vi "PublicAlarms.vi"(0 "reference in":refnum<class "Logger.lvclass">, 11 "error in (no error)":errorcluster, 13 "SV_Publisher in":refnum<class "SV_Publisher.lvclass">) -> (4 "reference out":refnum<class "Logger.lvclass">, 15 "error out":errorcluster)   [LabVIEW 2019, in "Logger.lvclass"]
uses:
  Logger.lvclass
  SV_Puplisher_class/SV_Publisher.lvclass
  Current Alarms.ctl
  EventData.ctl
  TypeDef/AlarmType.ctl
  Logger.lvclass/Logger.ctl
  SV_Puplisher_class/SV_Publisher.lvclass/SV_Publisher.ctl
  SV_Puplisher_class/Set SV.vi/1ae5d02c-efd0-450a-8aa4-8388e25d05bc.vi
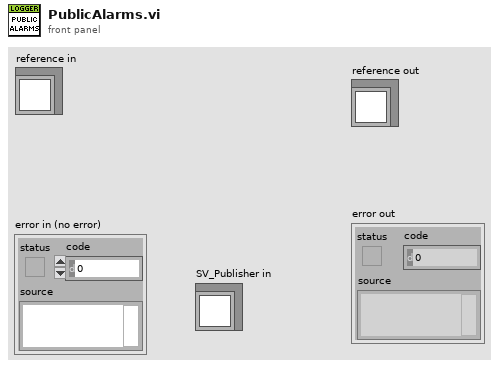
[diagram p1: front panel]
types:
  T1 = typedef "Logger.lvclass/Current Alarms.ctl" = cluster{"alarms":T2[]}
  T2 = typedef "Logger.lvclass/EventData.ctl" = cluster{"obj_tag":string, "event_tag":string, "Description":string, "ALARM TYPE":T3, "Value DBL":dbl, "Value INT":i32, "Value STR":string, "Time Stamp":timestamp}
  T3 = typedef "AlarmType.ctl" = enum16{"Normal", "Warning", "Alarm"}
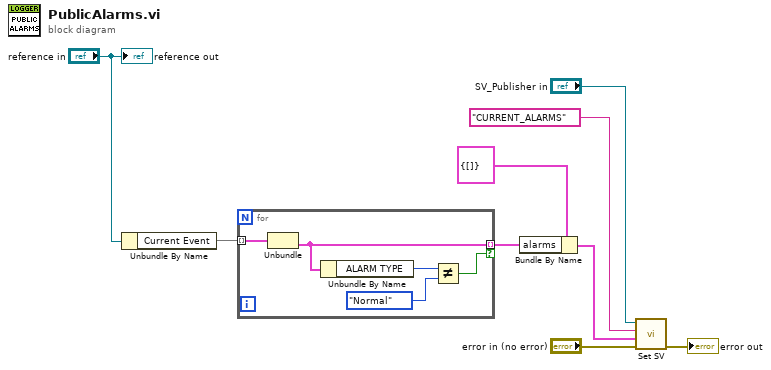
[diagram p0: block diagram]
diagram:
  n1 = Unbundle By Name("reference in") -> ("Current Event"=w3:map{string, T2})
  n2 = for {
    tunnel: w3 -> [w14] mode=indexing
    tunnel: [w13] -> w9 mode=indexing if=w10
    n3 = Unbundle(w14) -> ("Event"=w13:T2)  [unwired: 1 out]
    n4 = Unbundle By Name(w13) -> ("ALARM TYPE"=w12:T3)
    n5 = Not Equal?(x=w12, y=AlarmType."Normal") -> (x != y?=w10:bool)
  }
  n6 = Bundle By Name(cluster=T1 {"alarms"=[]} ("Current Alarms"), "alarms"=w9) -> (w8:T1)
  n7 = call "Set SV.vi"("error in (no error)"="error in (no error)", "SV Value"=w8, "SV Name"="CURRENT_ALARMS", "SV_Publisher in"="SV_Publisher in") -> ("error out"=→"error out":errorcluster)  [unwired: 6 in, 1 out]
  "reference out" <- "reference in"
